vi "Teleop.vi"(10 "Match Info":T1={"Autonomous Elapsed Seconds"=0.0, "TeleOp Elapsed Seconds"=0.0, "Disabled Elapsed Seconds"=0.0, "Visited Autonomous"=FALSE, "Visited TeleOp"=FALSE, "Visited Disabled"=FALSE, "Autonomous Settings"={"Autonomous Style"=enum."Independent", "VI Refnum"=refnum}}, 11 "Call Context":T2) -> ()   [LabVIEW 2017]
doc: "This VI is called for each TeleOp packet received from the DS where the robot is not disabled. It is often used to read from the joysticks and update I/O or to update setpoints for timed control loops. It should complete and return within 20 milliseconds or it may miss DS packets."
uses:
  <vilib>/Rock Robotics/WPI/DriverStation/WPI_DriverStationDerivedRobotMode.ctl
  <vilib>/Rock Robotics/WPI/DriverStation/WPI_DriverStationMatch Info.ctl
  <vilib>/Rock Robotics/WPI/Utilities/WPI_GetSetVariantRefNum.vi
  <vilib>/Rock Robotics/Network Tables/NT Write Boolean Array.vi
  <vilib>/Rock Robotics/Network Tables/NT Write Numeric Array.vi
  <vilib>/Rock Robotics/Network Tables/NT Read Boolean.vi
  <vilib>/Rock Robotics/Network Tables/NT Read Number.vi
  Robot Global Data.vi
panel:
  out "Sample Slider 0":dbl(slide) scale=0.0..5.0
  out "Sample Boolean 1":bool
  out "Sample Boolean 0":bool
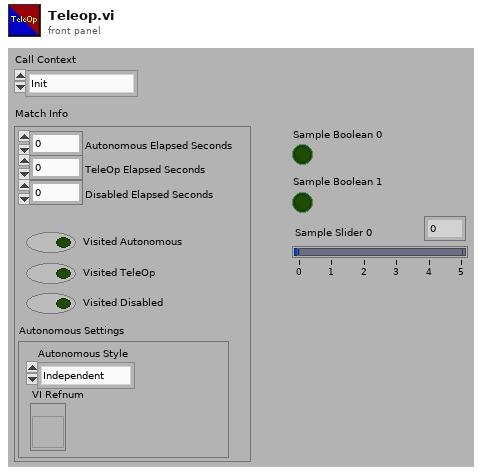
[diagram p1: front panel]
types:
  T1 = typedef "WPI_DriverStationMatch Info.ctl" = cluster{"Autonomous Elapsed Seconds":dbl, "TeleOp Elapsed Seconds":dbl, "Disabled Elapsed Seconds":dbl, "Visited Autonomous":bool, "Visited TeleOp":bool, "Visited Disabled":bool, "Autonomous Settings":cluster{"Autonomous Style":enum16{"Iterative", "Independent"}, "VI Refnum":refnum<vi>}}
  T2 = typedef "WPI_DriverStationDerivedRobotMode.ctl" = enum16{"Init", "Execute", "Stop"}
  T3 = typedef "WPI_MotorControlDeviceRef.ctl" = cluster{"DeviceStatus":errorcluster, "Type":T4, "PWM":cluster{"PWM Channel":T5, "DeadBand":T6}, "CAN":cluster{"Device Number":u8, "SetOutput VI Ref":variant, "GetOutput VI Ref":variant, "Enable VI Ref":variant, "Disable VI Ref":variant, "Data":variant}, "Invert":bool, "DIO PWM":cluster{"PWM \"Enable\" Channel":T5, "DIOChannel":T7, "PWM Rate":dbl}}
  T4 = typedef "WPI_MotorControlType.ctl" = enum16{"PWM", "CAN", "DIO PWM"}
  T5 = typedef "FPGA_DIOPWMChannel.ctl" = enum8{"PWM 0", "PWM 1", "PWM 2", "PWM 3", "PWM 4", "PWM 5", "PWM 6", "PWM 7", "PWM 8", "PWM 9", "PWM MXP 0", "PWM MXP 1", "PWM MXP 2", "PWM MXP 3", "PWM MXP 4", "PWM MXP 5", "PWM MXP 6", "PWM MXP 7", "PWM MXP 8", "PWM MXP 9", "Invalid"}
  T6 = typedef "WPI_PWMDeadband.ctl" = cluster{"Name":string, "maxPositivePwm":i32, "minPositivePwm":i32, "centerPwm":i32, "maxNegativePwm":i32, "minNegativePwm":i32, "angularRange":u16}
  T7 = typedef "FPGA_DIOChannel.ctl" = enum8{"DIO 0", "DIO 1", "DIO 2", "DIO 3", "DIO 4", "DIO 5", "DIO 6", "DIO 7", "DIO 8", "DIO 9", "DIO MXP 0", "DIO MXP 1", "DIO MXP 2", "DIO MXP 3", "DIO MXP 4", "DIO MXP 5", "DIO MXP 6", "DIO MXP 7", "DIO MXP 8", "DIO MXP 9", "DIO MXP 10", "DIO MXP 11", "DIO MXP 12", "DIO MXP 13", "DIO MXP 14", "DIO MXP 15", "SPI Port CS1", "SPI Port CS2", "SPI Port CS3", "SPI Port MISO", "SPI Port MOSI", "Invalid"}
  T8 = typedef "WPI_RobotDriveDevRef.ctl" = cluster{"DevStatus":errorcluster, "Motors[]":T3[], "Square Inputs":bool, "Max Output":dbl}
  T9 = typedef "WPI_JoystickDevRef.ctl" = cluster{"Device":T10}
  T10 = typedef "WPI_JoystickDeviceEnum.ctl" = enum16{"USB 0", "USB 1", "USB 2", "USB 3", "USB 4", "USB 5"}
  T11 = typedef "WPI_CompressorDevRef.ctl" = cluster{"DevStatus":errorcluster, "Pneumatics Control Module":u8}
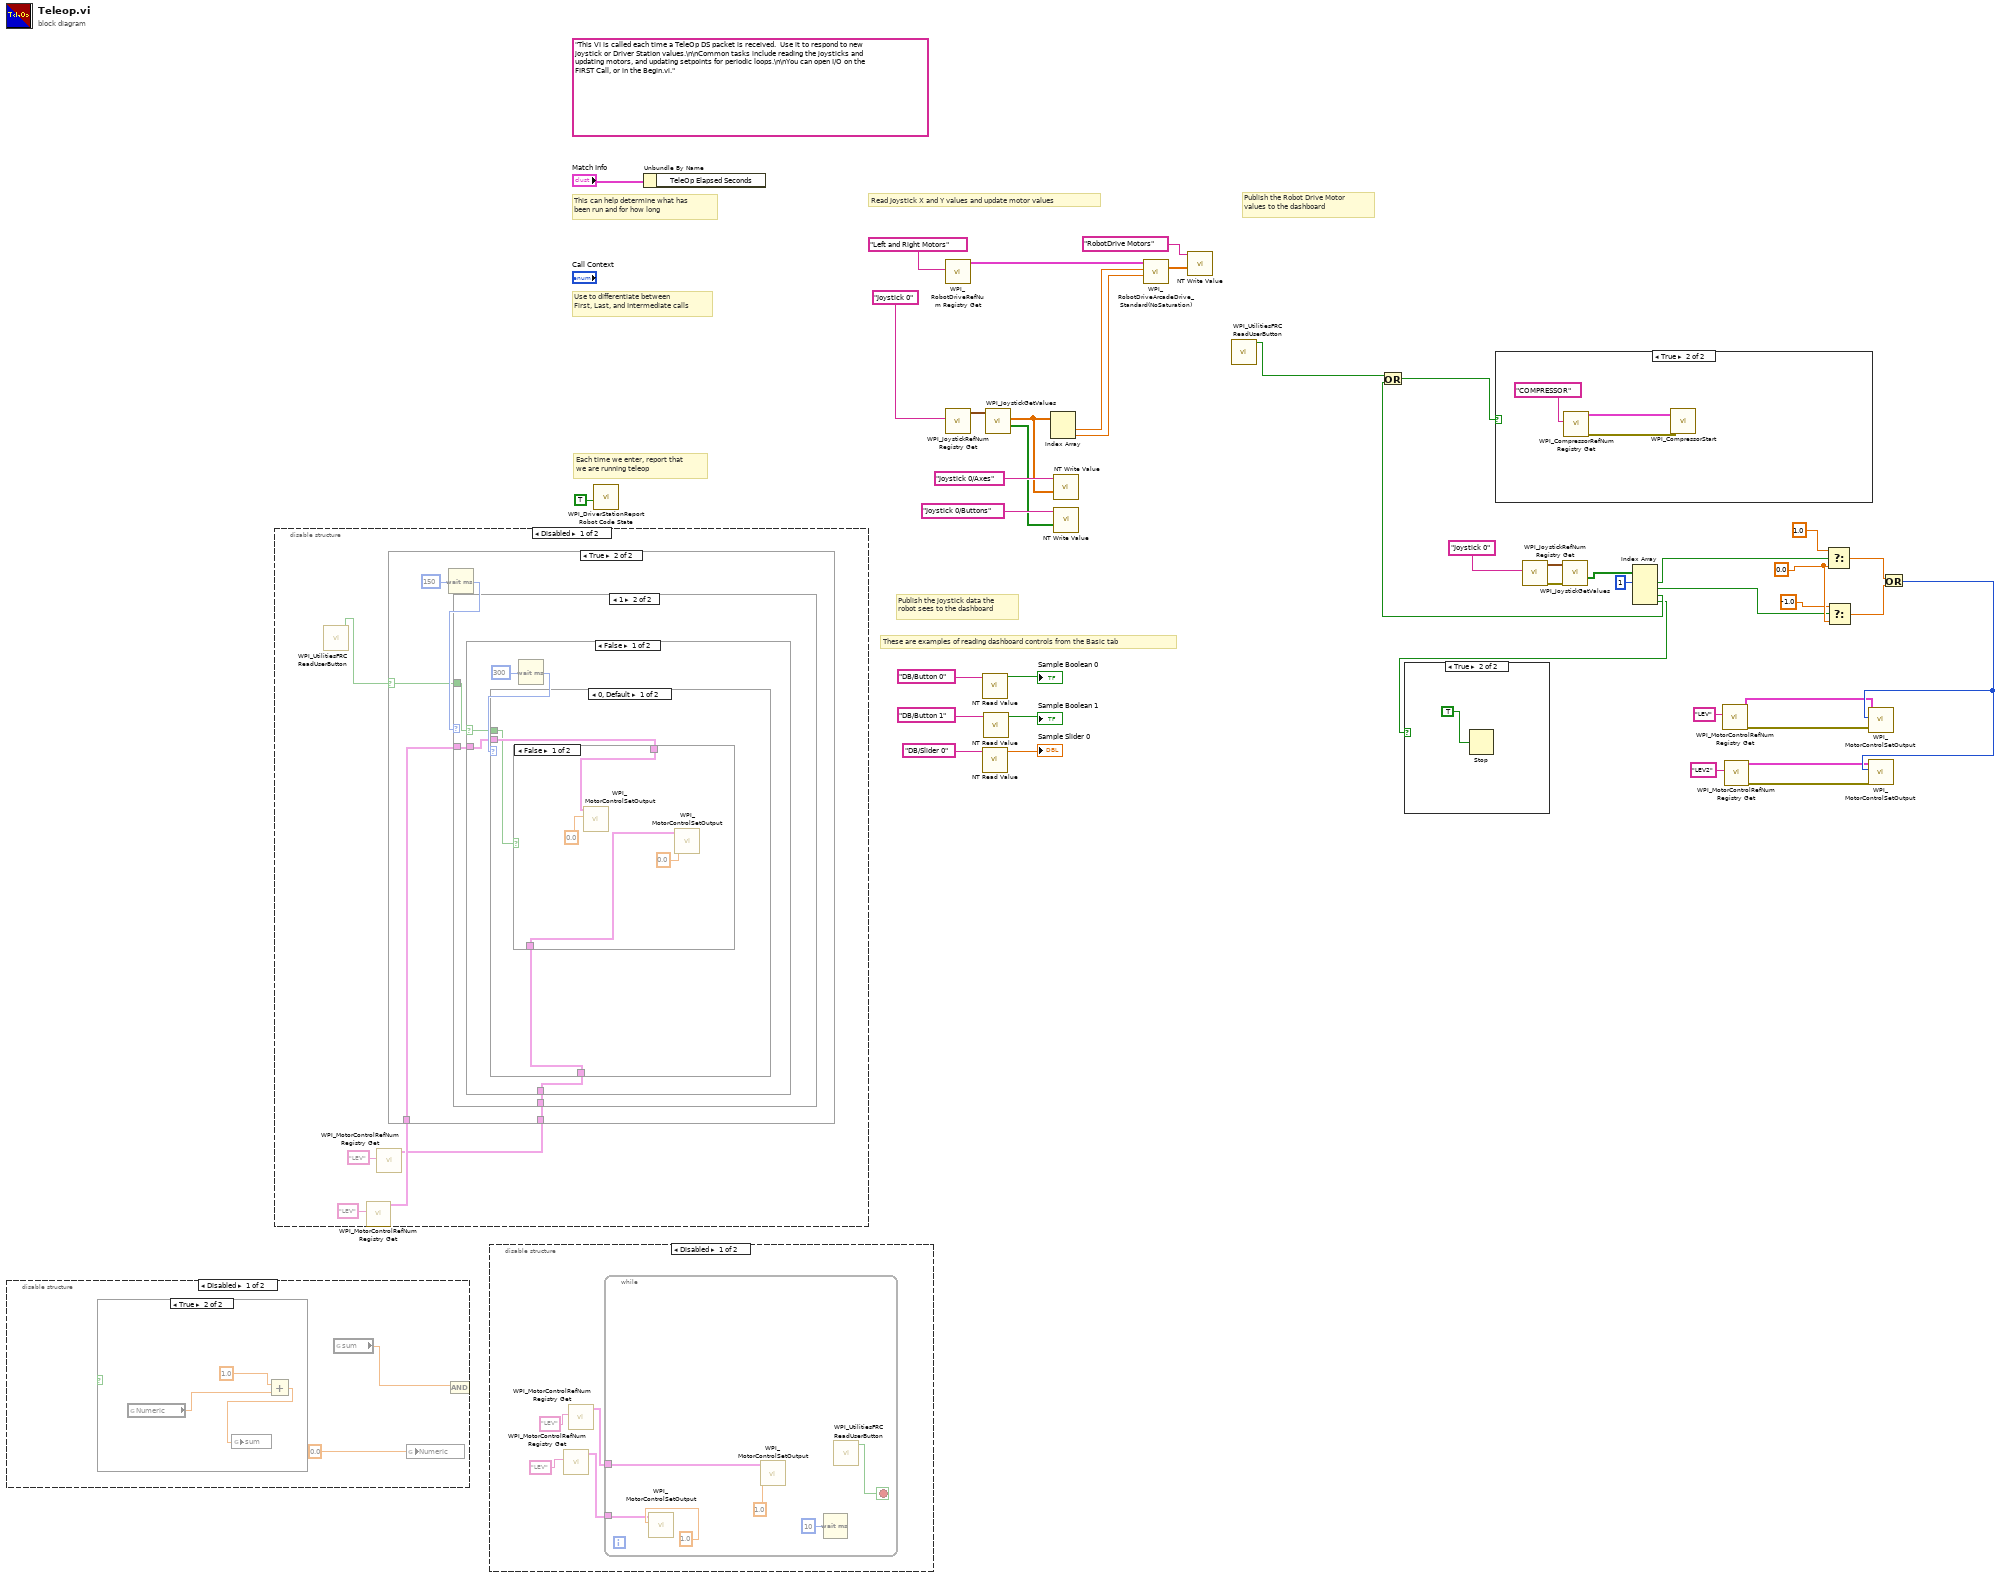
[diagram p0: block diagram]
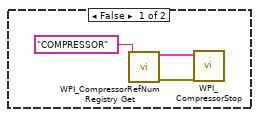
[diagram p3: hidden frame]
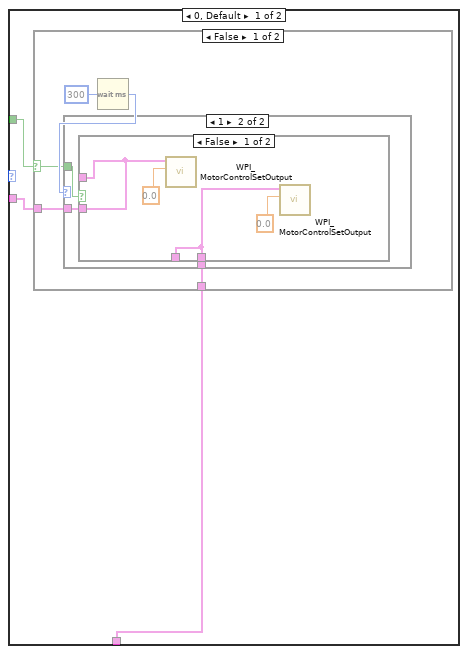
[diagram p8: hidden frame]
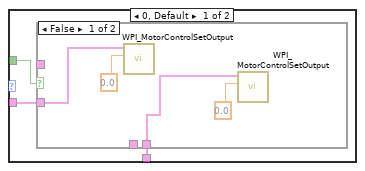
[diagram p9: hidden frame]
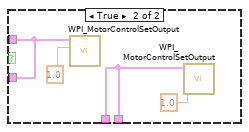
[diagram p10: hidden frame]
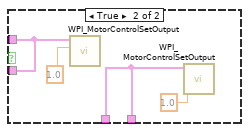
[diagram p11: hidden frame]
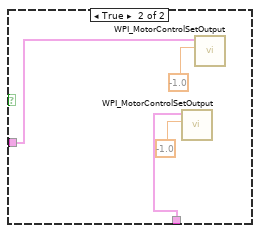
[diagram p12: hidden frame]
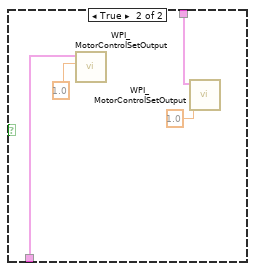
[diagram p13: hidden frame]
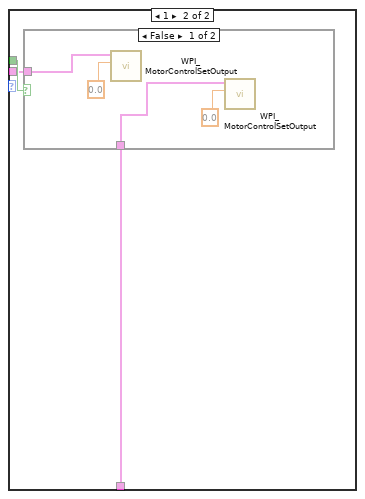
[diagram p14: hidden frame]
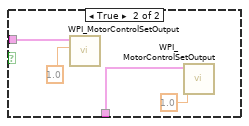
[diagram p15: hidden frame]
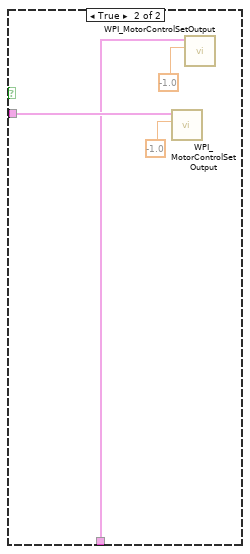
[diagram p16: hidden frame]
diagram:
  w18 = 0.0 ("t")
  (unwired) "This VI is called each time a TeleOp DS packet is received.  Use it to respond to new joystick or Driver Station values.\n\nCommon tasks include reading the joysticks and updating motors, and updating setpoints for periodic loops.\n\nYou can open I/O on the FIRST Call, or in the Begin.vi."
  # "Publish the Robot Drive Motor\nvalues to the dashboard"
  # "These are examples of reading dashboard controls from the Basic tab"
  # "Publish the joystick data the\nrobot sees to the dashboard"
  # "Each time we enter, report that\nwe are running teleop"
  # "Use to differentiate between\nFirst, Last, and Intermediate calls"
  # "This can help determine what has\nbeen run and for how long"
  # "Read Joystick X and Y values and update motor values"
  n1 = disable-structure shown="Disabled" {
    frame Disabled {
      n2 = case shown="True" {
        selector: _ -> [_ _]
        frame False {
        }
        frame True {
          n3 = global read "Robot Global Data.vi" "Numeric"() -> (w48:dbl)
          n4 = Add(x=1.0 ("Numeric"), y=w48) -> (x+y=w46:dbl)
          n5 = global write "Robot Global Data.vi" "sum"(w46) -> ()
        }
      }
      n6 = global read "Robot Global Data.vi" "sum"() -> (w44:dbl)
      n7 = global write "Robot Global Data.vi" "Numeric"(0.0 ("Numeric")) -> ()
      n8 = And(x=w44) -> ()  [unwired: 1 in, 1 out]
    }
    frame Enabled {
    }
  }
  n9 = disable-structure shown="Disabled" {
    frame Disabled {
      n10 = call <vilib>:"WPI_UtilitiesFRC ReadUserButton.vi"() -> ("User Button"=w53:bool)  [unwired: 10 in, 1 out]
      n11 = call <vilib>:"WPI_MotorControlRefNum Registry Get.vi"("refnum name"="LEV") -> ("MotorControlDevRef"=w50:T3)  [unwired: 9 in, 1 out]
      n12 = call <vilib>:"WPI_MotorControlRefNum Registry Get.vi"("refnum name"="LEV") -> ("MotorControlDevRef"=w49:T3)  [unwired: 9 in, 1 out]
      n13 = case shown="True" w53 {
        selector: w53 -> [_ w56]
        tunnel: w50 -> [_ w55]
        tunnel: w49 -> [_ w54]
        frame False {
        }
        frame True {
          n14 = Wait (ms)(milliseconds to wait=u32 150) -> (millisecond timer value=w58:u32)
          n15 = case shown="1" w58 {
            tunnel: w56 -> [w59 w95]
            tunnel: w55 -> [w61 w94]
            tunnel: w54 -> [w60 w93]
            frame 0, Default {
              n16 = case shown="False" w59 {
                selector: w59 -> [w64 _]
                tunnel: w61 -> [w63 w90]
                tunnel: w60 -> [w62 w89]
                frame False {
                  n17 = Wait (ms)(milliseconds to wait=u32 300) -> (millisecond timer value=w65:u32)
                  n18 = case shown="1" w65 {
                    tunnel: w64 -> [w69 w80]
                    tunnel: w63 -> [w68 w79]
                    tunnel: w62 -> [w67 w78]
                    frame 0, Default {
                      n19 = case shown="False" w69 {
                        tunnel: [_ w75] -> _
                        tunnel: [_ w74] -> _
                        tunnel: w68 -> [w71 w75]
                        tunnel: w67 -> [w70 w74]
                        frame False {
                          n20 = call <vilib>:"WPI_MotorControlSetOutput.vi"("Output"=0.0, "MotorControlDevRef"=w71) -> ()  [unwired: 7 in, 3 out]
                          n21 = call <vilib>:"WPI_MotorControlSetOutput.vi"("Output"=0.0, "MotorControlDevRef"=w70) -> ()  [unwired: 7 in, 3 out]
                        }
                        frame True {
                          n22 = call <vilib>:"WPI_MotorControlSetOutput.vi"("Output"=1.0, "MotorControlDevRef"=w75) -> ()  [unwired: 7 in, 3 out]
                          n23 = call <vilib>:"WPI_MotorControlSetOutput.vi"("Output"=1.0, "MotorControlDevRef"=w74) -> ()  [unwired: 7 in, 3 out]
                        }
                      }
                    }
                    frame 1 {
                      n24 = case shown="False" w80 {
                        tunnel: [w82 w85] -> _
                        tunnel: [w81 w86] -> _
                        tunnel: w79 -> [w82 w85]
                        tunnel: w78 -> [w81 w86]
                        frame False {
                          n25 = call <vilib>:"WPI_MotorControlSetOutput.vi"("Output"=0.0, "MotorControlDevRef"=w82) -> ()  [unwired: 7 in, 3 out]
                          n26 = call <vilib>:"WPI_MotorControlSetOutput.vi"("Output"=0.0, "MotorControlDevRef"=w81) -> ()  [unwired: 7 in, 3 out]
                        }
                        frame True {
                          n27 = call <vilib>:"WPI_MotorControlSetOutput.vi"("Output"=1.0, "MotorControlDevRef"=w85) -> ()  [unwired: 7 in, 3 out]
                          n28 = call <vilib>:"WPI_MotorControlSetOutput.vi"("Output"=1.0, "MotorControlDevRef"=w86) -> ()  [unwired: 7 in, 3 out]
                        }
                      }
                    }
                  }
                }
                frame True {
                  n29 = call <vilib>:"WPI_MotorControlSetOutput.vi"("Output"=-1.0, "MotorControlDevRef"=w89) -> ()  [unwired: 7 in, 3 out]
                  n30 = call <vilib>:"WPI_MotorControlSetOutput.vi"("Output"=-1.0, "MotorControlDevRef"=w90) -> ()  [unwired: 7 in, 3 out]
                }
              }
            }
            frame 1 {
              n31 = case shown="False" w95 {
                selector: w95 -> [w98 _]
                tunnel: w94 -> [w97 w125]
                tunnel: w93 -> [w96 w123]
                frame False {
                  n32 = Wait (ms)(milliseconds to wait=u32 300) -> (millisecond timer value=w99:u32)
                  n33 = case shown="0, Default" w99 {
                    tunnel: w98 -> [w101 w114]
                    tunnel: w97 -> [w102 w113]
                    tunnel: w96 -> [w103 w112]
                    frame 0, Default {
                      n34 = case shown="False" w101 {
                        tunnel: w103 -> [w105 w109]
                        tunnel: w102 -> [w104 w108]
                        frame False {
                          n35 = call <vilib>:"WPI_MotorControlSetOutput.vi"("Output"=0.0, "MotorControlDevRef"=w104) -> ()  [unwired: 7 in, 3 out]
                          n36 = call <vilib>:"WPI_MotorControlSetOutput.vi"("Output"=0.0, "MotorControlDevRef"=w105) -> ()  [unwired: 7 in, 3 out]
                        }
                        frame True {
                          n37 = call <vilib>:"WPI_MotorControlSetOutput.vi"("Output"=1.0, "MotorControlDevRef"=w109) -> ()  [unwired: 7 in, 3 out]
                          n38 = call <vilib>:"WPI_MotorControlSetOutput.vi"("Output"=1.0, "MotorControlDevRef"=w108) -> ()  [unwired: 7 in, 3 out]
                        }
                      }
                    }
                    frame 1 {
                      n39 = case shown="False" w114 {
                        tunnel: w113 -> [w115 w120]
                        tunnel: w112 -> [w116 w119]
                        frame False {
                          n40 = call <vilib>:"WPI_MotorControlSetOutput.vi"("Output"=0.0, "MotorControlDevRef"=w115) -> ()  [unwired: 7 in, 3 out]
                          n41 = call <vilib>:"WPI_MotorControlSetOutput.vi"("Output"=0.0, "MotorControlDevRef"=w116) -> ()  [unwired: 7 in, 3 out]
                        }
                        frame True {
                          n42 = call <vilib>:"WPI_MotorControlSetOutput.vi"("Output"=1.0, "MotorControlDevRef"=w120) -> ()  [unwired: 7 in, 3 out]
                          n43 = call <vilib>:"WPI_MotorControlSetOutput.vi"("Output"=1.0, "MotorControlDevRef"=w119) -> ()  [unwired: 7 in, 3 out]
                        }
                      }
                    }
                  }
                }
                frame True {
                  n44 = call <vilib>:"WPI_MotorControlSetOutput.vi"("Output"=-1.0, "MotorControlDevRef"=w125) -> ()  [unwired: 7 in, 3 out]
                  n45 = call <vilib>:"WPI_MotorControlSetOutput.vi"("Output"=-1.0, "MotorControlDevRef"=w123) -> ()  [unwired: 7 in, 3 out]
                }
              }
            }
          }
        }
      }
    }
    frame Enabled {
    }
  }
  n46 = disable-structure shown="Disabled" {
    frame Disabled {
      n47 = call <vilib>:"WPI_MotorControlRefNum Registry Get.vi"("refnum name"="LEV") -> ("MotorControlDevRef"=w127:T3)  [unwired: 9 in, 1 out]
      n48 = call <vilib>:"WPI_MotorControlRefNum Registry Get.vi"("refnum name"="LEV") -> ("MotorControlDevRef"=w128:T3)  [unwired: 9 in, 1 out]
      n49 = while {
        tunnel: w128 -> [w133]
        tunnel: w127 -> [w132]
        stop <- w136 stop-if-true
        n50 = call <vilib>:"WPI_MotorControlSetOutput.vi"("Output"=1.0, "MotorControlDevRef"=w132) -> ()  [unwired: 7 in, 3 out]
        n51 = call <vilib>:"WPI_MotorControlSetOutput.vi"("Output"=1.0, "MotorControlDevRef"=w133) -> ()  [unwired: 7 in, 3 out]
        n52 = Wait (ms)(milliseconds to wait=u32 10) -> ()  [unwired: 1 out]
        n53 = call <vilib>:"WPI_UtilitiesFRC ReadUserButton.vi"() -> ("User Button"=w136:bool)  [unwired: 10 in, 1 out]
      }
    }
    frame Enabled {
    }
  }
  n54 = call <vilib>:"WPI_DriverStationReport Robot Code State.vi"("TeleOp"=TRUE ("Autonomous")) -> ()  [unwired: 10 in, 1 out]
  n55 = Unbundle By Name("Match Info") -> ()  [unwired: 1 out]
  n56 = call <vilib>:"WPI_RobotDriveRefNum Registry Get.vi"("refnum name"="Left and Right Motors") -> ("RobotDriveDevRef"=w41:T8)  [unwired: 1 in, 9 out]
  n57 = call <vilib>:"WPI_JoystickRefNum Registry Get.vi"("refnum name"="Joystick 0") -> ("JoystickDevRef"=w38:T9)  [unwired: 1 in, 9 out]
  n58 = call-poly <vilib>:"NT Read Value.vi"("Name"="DB/Button 0" ("refnum name")) -> ("Boolean"=→"Sample Boolean 0":bool)  [unwired: 9 in, 1 out]
  n59 = call-poly <vilib>:"NT Read Value.vi"("Name"="DB/Slider 0" ("refnum name")) -> ("Numeric"=→"Sample Slider 0":dbl)  [unwired: 9 in, 1 out]
  n60 = call-poly <vilib>:"NT Read Value.vi"("Name"="DB/Button 1" ("refnum name")) -> ("Boolean"=→"Sample Boolean 1":bool)  [unwired: 9 in, 1 out]
  n61 = call <vilib>:"WPI_JoystickGetValues.vi"("JoystickDevRef"=w38) -> ("Buttons"=w2:bool[], "Axes"=w33:dbl[])  [unwired: 6 in, 3 out]
  n62 = Index Array(array=w33) -> (element #1=w40:dbl, element #2=w36:dbl)  [unwired: 2 in]
  n63 = call-poly <vilib>:"NT Write Value.vi"("Numeric Array"=w33, "Name"="Joystick 0/Axes") -> ()  [unwired: 9 in, 1 out]
  n64 = call-poly <vilib>:"NT Write Value.vi"("Boolean Array"=w2, "Name"="Joystick 0/Buttons") -> ()  [unwired: 9 in, 1 out]
  n65 = call <vilib>:"WPI_RobotDriveArcadeDrive_Standard(NoSaturation).vi"("Y axis value"=w36, "X axis value"=w40, "RobotDriveDevRef"=w41) -> ("Motor Values"=w26:dbl[])  [unwired: 1 in, 7 out]
  n66 = call-poly <vilib>:"NT Write Value.vi"("Numeric Array"=w26, "Name"="RobotDrive Motors") -> ()  [unwired: 9 in, 1 out]
  n67 = call <vilib>:"WPI_UtilitiesFRC ReadUserButton.vi"() -> ("User Button"=w5:bool)  [unwired: 10 in, 1 out]
  n68 = call <vilib>:"WPI_JoystickRefNum Registry Get.vi"("refnum name"="Joystick 0") -> ("error out"=w21:errorcluster, "JoystickDevRef"=w24:T9)  [unwired: 1 in, 8 out]
  n69 = call <vilib>:"WPI_JoystickGetValues.vi"("error in (no error)"=w21, "JoystickDevRef"=w24) -> ("Buttons"=w22:bool[])  [unwired: 5 in, 4 out]
  n70 = Index Array(array=w22, index #1=1 ("index")) -> (element #1=w7:bool, element #2=w6:bool, element #3=w4:bool, element #4=w1:bool)  [unwired: 3 in]
  n71 = Or(x=w5, y=w4) -> (x .or. y?=w3:bool)
  n72 = case shown="True" w1 {
    frame False {
    }
    frame True {
      n73 = Stop(stop? (T)=TRUE) -> ()
    }
  }
  n74 = case shown="True" w3 {
    frame False {
      n75 = call <vilib>:"WPI_CompressorRefNum Registry Get.vi"("refnum name"="COMPRESSOR") -> ("error out"=w140:errorcluster, "CompressorDevRef"=w139:T11)  [unwired: 9 in]
      n76 = call <vilib>:"WPI_CompressorStop.vi"("error in (no error)"=w140, "CompressorDevRef"=w139) -> ()  [unwired: 8 in, 2 out]
    }
    frame True {
      n77 = call <vilib>:"WPI_CompressorRefNum Registry Get.vi"("refnum name"="COMPRESSOR") -> ("error out"=w141:errorcluster, "CompressorDevRef"=w142:T11)  [unwired: 9 in]
      n78 = call <vilib>:"WPI_CompressorStart.vi"("error in (no error)"=w141, "CompressorDevRef"=w142) -> ()  [unwired: 8 in, 2 out]
    }
  }
  n79 = call <vilib>:"WPI_MotorControlRefNum Registry Get.vi"("refnum name"="LEV") -> ("error out"=w11:errorcluster, "MotorControlDevRef"=w10:T3)  [unwired: 9 in]
  n80 = call <vilib>:"WPI_MotorControlRefNum Registry Get.vi"("refnum name"="LEV2") -> ("error out"=w12:errorcluster, "MotorControlDevRef"=w13:T3)  [unwired: 9 in]
  n81 = Select(t=1.0, s=w7, f=w18) -> (s? t:f=w16:dbl)
  n82 = Select(t=-1.0, s=w6, f=w18) -> (s? t:f=w15:dbl)
  n83 = Or(x=w16, y=w15) -> (x .or. y?=w14:i32)
  n84 = call <vilib>:"WPI_MotorControlSetOutput.vi"("error in (no error)"=w11, "Output"=w14, "MotorControlDevRef"=w10) -> ()  [unwired: 6 in, 3 out]
  n85 = call <vilib>:"WPI_MotorControlSetOutput.vi"("error in (no error)"=w12, "Output"=w14, "MotorControlDevRef"=w13) -> ()  [unwired: 6 in, 3 out]
